vi "Simulated_Tank_Drive.vi"   [LabVIEW 2012]
uses:
  State_Machine_Enum.ctl
  <vilib>/Rock Robotics/WPI/RobotDrive/WPI_RobotDriveGetSetRefNum.vi
  Robot Global Data.vi
types:
  T1 = typedef "State_Machine_Enum.ctl" = enum16{"Idle", "Start", "Do", "Stop", "Init"}
  T2 = typedef "WPI_RobotDriveDevRef.ctl" = cluster{"DevStatus":errorcluster, "Motors[]":T3[], "Square Inputs":bool, "Max Output":dbl, "Isochronous":bool}
  T3 = typedef "WPI_MotorControlDeviceRef.ctl" = cluster{"DeviceStatus":errorcluster, "Type":enum16{"PWM", "CAN"}, "PWM":cluster{"Digital Module":T4, "PWM Channel":T5, "DeadBand":T6}, "CAN":cluster{"Device Number":u8, "Control Mode":T7, "Semaphore":T8, "Max Vout":dbl}, "Invert":bool, "TransformRef":T9, "InvTransformRef":T9}
  T4 = typedef "FPGA_TypedefDigitalModule.ctl" = enum16{"Digital Module 1", "Digital Module 2"}
  T5 = typedef "FPGA_DIOPWMChannel.ctl" = enum8{"PWM 1", "PWM 2", "PWM 3", "PWM 4", "PWM 5", "PWM 6", "PWM 7", "PWM 8", "PWM 9", "PWM 10", "Invalid"}
  T6 = typedef "WPI_PWMDeadband.ctl" = cluster{"Name":string, "maxPositivePwm":i32, "minPositivePwm":i32, "centerPwm":i32, "maxNegativePwm":i32, "minNegativePwm":i32, "angularRange":u16}
  T7 = typedef "WPI_CANJaguar_ControlMode.ctl" = enum8{"Percent VBus", "Current", "Speed", "Position", "Voltage"}
  T8 = typedef "Semaphore RefNum" = refnum<k1>
  T9 = typedef "WPI_PWMTransform_ConPane.ctl" = refnum<vi>
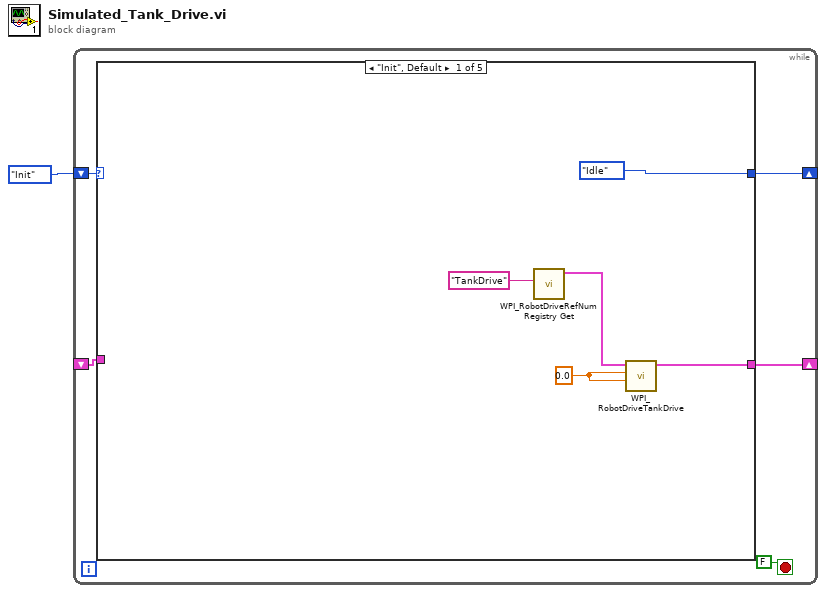
[diagram p0: block diagram]
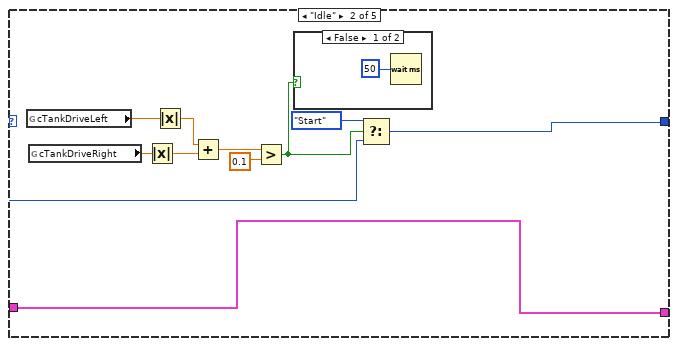
[diagram p2: hidden frame]
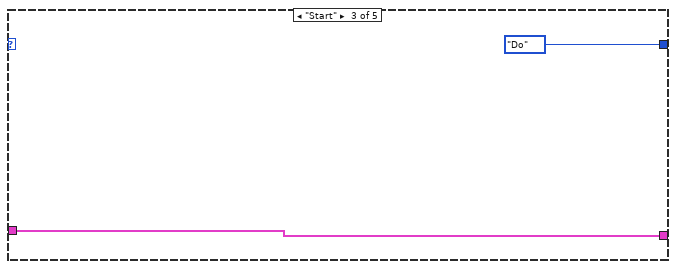
[diagram p4: hidden frame]
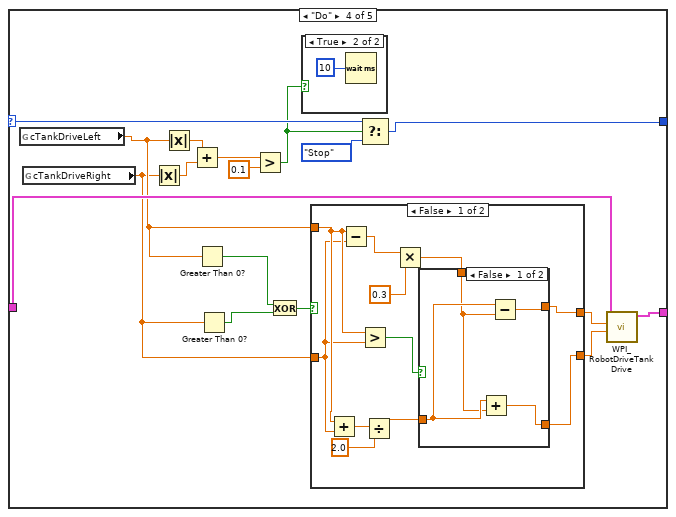
[diagram p5: hidden frame]
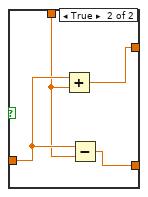
[diagram p6: hidden frame]
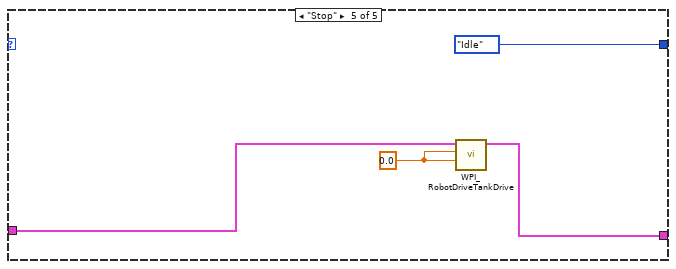
[diagram p9: hidden frame]
diagram:
  n1 = while {
    shift-right: [w4] -> _
    shift-left: State_Machine_Enum."Init" ("State") -> [w5]
    shift-right: [w3] -> _
    shift-left: _ -> [w2]
    stop <- FALSE stop-if-true
    n2 = case shown="\"Init\", Default" w5 {
      selector: w5 -> [_ w17 _ w38 _]
      tunnel: [State_Machine_Enum."Idle" ("State") w16 State_Machine_Enum."Do" ("State") w37 State_Machine_Enum."Idle" ("State")] -> w4
      tunnel: [w7 w12 w25 w35 w67] -> w3
      tunnel: w2 -> [_ w12 w25 w36 w66]
      frame "Init", Default {
        w9 = 0.0 ("Left axis value")
        n3 = call <vilib>:"WPI_RobotDriveRefNum Registry Get.vi"("refnum name"="TankDrive") -> ("RobotDriveDevRef"=w8:T2)  [unwired: 9 in, 1 out]
        n4 = call <vilib>:"WPI_RobotDriveTankDrive.vi"("Right axis value"=w9, "Left axis value"=w9, "RobotDriveDevRef"=w8) -> ("RobotDriveDevRef"=w7:T2)  [unwired: 6 in, 2 out]
      }
      frame "Idle" {
        n5 = global read "Robot Global Data.vi" "cTankDriveLeft"() -> (w15:dbl)
        n6 = global read "Robot Global Data.vi" "cTankDriveRight"() -> (w14:dbl)
        n7 = Absolute Value(x=w14) -> (abs(x)=w21:dbl)
        n8 = Absolute Value(x=w15) -> (abs(x)=w22:dbl)
        n9 = Add(x=w22, y=w21) -> (x+y=w20:dbl)
        n10 = Greater?(x=w20, y=0.1) -> (0:w18:bool)
        n11 = case shown="False" w18 {
          frame False {
            n12 = Wait (ms)(milliseconds to wait=u32 50) -> ()  [unwired: 1 out]
          }
          frame True {
          }
        }
        n13 = Select(t=State_Machine_Enum."Start" ("State"), s=w18, f=w17) -> (s? t:f=w16:T1)
      }
      frame "Start" {
      }
      frame "Do" {
        n14 = global read "Robot Global Data.vi" "cTankDriveLeft"() -> (w29:dbl)
        n15 = global read "Robot Global Data.vi" "cTankDriveRight"() -> (w28:dbl)
        n16 = Absolute Value(x=w28) -> (abs(x)=w41:dbl)
        n17 = Absolute Value(x=w29) -> (abs(x)=w42:dbl)
        n18 = Add(x=w42, y=w41) -> (x+y=w39:dbl)
        n19 = Greater Than 0?(x=w29) -> (x > 0?=w31:bool)
        n20 = Greater Than 0?(x=w28) -> (x > 0?=w30:bool)
        n21 = Greater?(x=w39, y=0.1) -> (0:w34:bool)
        n22 = Exclusive Or(1:w30, 2:w31) -> (0:w32:bool)
        n23 = case shown="True" w34 {
          frame False {
          }
          frame True {
            n24 = Wait (ms)(milliseconds to wait=u32 10) -> ()  [unwired: 1 out]
          }
        }
        n25 = case shown="False" w32 {
          tunnel: w28 -> [w45 w62]
          tunnel: [w48 w63] -> w26
          tunnel: [w47 w62] -> w27
          tunnel: w29 -> [w46 w63]
          frame False {
            n26 = Add(x=w46, y=w45) -> (x+y=w53:dbl)
            n27 = Subtract(x=w46, y=w45) -> (x-y=w51:dbl)
            n28 = Greater?(x=w46, y=w45) -> (0:w43:bool)
            n29 = Divide(x=w53, y=2.0) -> (x/y=w49:dbl)
            n30 = Multiply(x=w51, y=0.3) -> (x*y=w44:dbl)
            n31 = case shown="False" w43 {
              tunnel: w49 -> [w56 w60]
              tunnel: [w57 w61] -> w48
              tunnel: [w54 w58] -> w47
              tunnel: w44 -> [w55 w59]
              frame False {
                n32 = Add(x=w56, y=w55) -> (x+y=w54:dbl)
                n33 = Subtract(x=w56, y=w55) -> (x-y=w57:dbl)
              }
              frame True {
                n34 = Add(x=w60, y=w59) -> (x+y=w61:dbl)
                n35 = Subtract(x=w60, y=w59) -> (x-y=w58:dbl)
              }
            }
          }
          frame True {
          }
        }
        n36 = Select(t=w38, s=w34, f=State_Machine_Enum."Stop" ("State")) -> (s? t:f=w37:T1)
        n37 = call <vilib>:"WPI_RobotDriveTankDrive.vi"("Right axis value"=w27, "Left axis value"=w26, "RobotDriveDevRef"=w36) -> ("RobotDriveDevRef"=w35:T2)  [unwired: 6 in, 2 out]
      }
      frame "Stop" {
        w68 = 0.0 ("Left axis value")
        n38 = call <vilib>:"WPI_RobotDriveTankDrive.vi"("Right axis value"=w68, "Left axis value"=w68, "RobotDriveDevRef"=w66) -> ("RobotDriveDevRef"=w67:T2)  [unwired: 6 in, 2 out]
      }
    }
  }
